vi "VectorNorm.vi"(0 "Vector":dbl[](array[numeric])) -> (1 "Unit Vector":dbl[](array[numeric]), 2 "Norm":dbl)   [LabVIEW 2014, in "ForceField.lvclass"]
uses:
  ForceField.lvclass
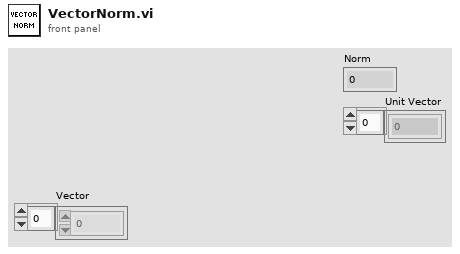
[diagram p1: front panel]
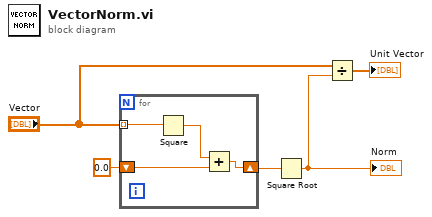
[diagram p0: block diagram]
diagram:
  n1 = for {
    tunnel: "Vector" -> [w9] mode=indexing
    shift-right: [w7] -> w4
    shift-left: 0.0 -> [w6]
    n2 = Square(x=w9) -> (x^2=w8:dbl)
    n3 = Add(x=w8, y=w6) -> (x+y=w7:dbl)
  }
  n4 = Square Root(x=w4) -> (sqrt(x)=w3:dbl)
  "Norm" <- w3
  n5 = Divide(x="Vector", y=w3) -> (x/y=→"Unit Vector":dbl[])
